vi "Time Count.vi"(10 "Action":enum16{"Count", "Stop", "Reset"}(ring)) -> (2 "Time":dbl)   [LabVIEW 2014]
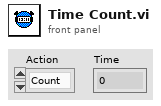
[diagram p1: front panel]
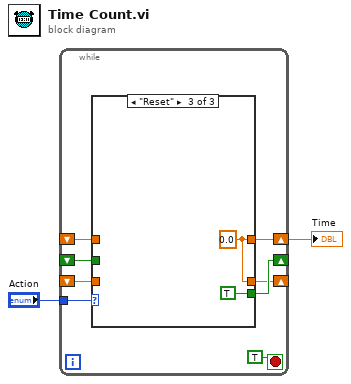
[diagram p0: block diagram]
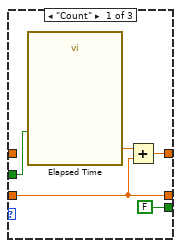
[diagram p2: hidden frame]
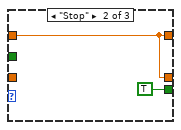
[diagram p3: hidden frame]
diagram:
  n1 = while {
    shift-right: [w10] -> w1
    shift-left: _ -> [w8]
    tunnel: "Action" -> [w9]
    shift-right: [w5] -> _
    shift-left: _ -> [w6]
    shift-right: [w3] -> _
    shift-left: _ -> [w4]
    stop <- TRUE stop-if-true
    n2 = case shown="\"Reset\"" w9 {
      tunnel: [w13 w16 w18] -> w10
      tunnel: w8 -> [_ w16 _]
      tunnel: w6 -> [w14 _ _]
      tunnel: [FALSE TRUE TRUE] -> w5
      tunnel: w4 -> [w12 _ _]
      tunnel: [w12 w16 w18] -> w3
      frame "Count" {
        n3 = call "Elapsed Time"("Reset"=w14) -> ("Elapsed Time (s)"=w15:dbl)  [unwired: 11 in, 7 out]
        n4 = Add(x=w15, y=w12) -> (x+y=w13:dbl)
      }
      frame "Stop" {
      }
      frame "Reset" {
        w18 = 0.0 ("Elapsed Time (s)")
      }
    }
  }
  "Time" <- w1
